vi "JL_Get_Latest_Build_From_Artifactory.vi"(0 "Repository":string="CIBuild", 11 "Error In":errorcluster) -> (4 "Output Path":path, 6 "Build":string, 15 "Error Out":errorcluster)   [LabVIEW 2019]
uses:
  <vilib>/regexp/Match Regular Expression.xnode
  <vilib>/httpClient/LabVIEWHTTPClient.lvlib
  <vilib>/zip/NI_Unzip.lvlib
panel:
  out "Numeric":i32
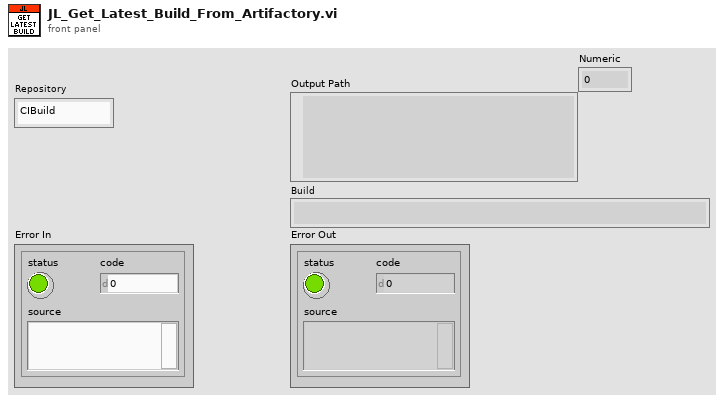
[diagram p1: front panel]
types:
  T1 = typedef "LabVIEWHTTPClient.lvlib/ClientHandle.ctl" = refnum<k1>
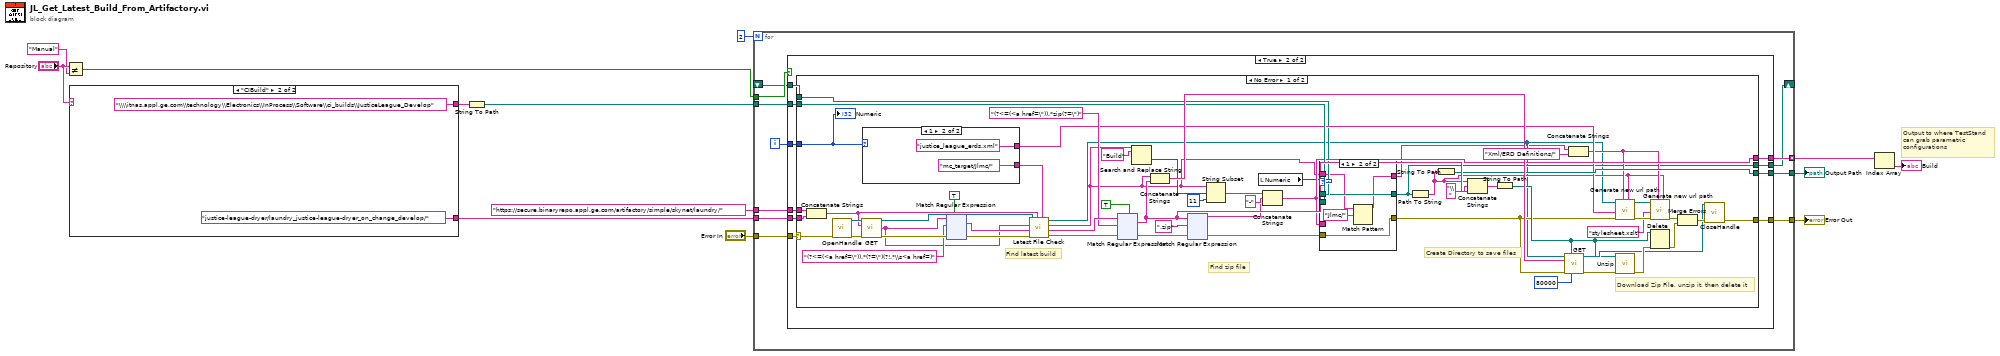
[diagram p0: block diagram]
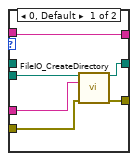
[diagram p3: hidden frame]
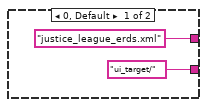
[diagram p4: hidden frame]
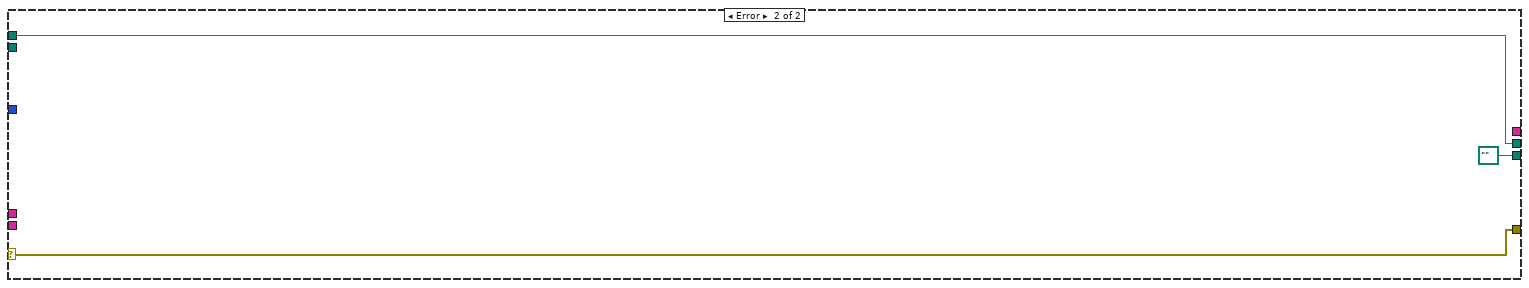
[diagram p5: hidden frame]
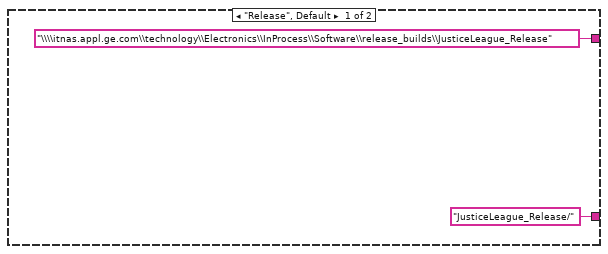
[diagram p6: hidden frame]
diagram:
  # "Output to where TestStand\ncan grab parametric\nconfigurations"
  n1 = Not Equal?(x="Repository", y="Manual") -> (x != y?=w12:bool)
  n2 = case shown="\"CIBuild\"" "Repository" {
    tunnel: ["\\\\itnas.appl.ge.com\\technology\\Electronics\\InProcess\\Software\\release_builds\\JusticeLeague_Release" "\\\\itnas.appl.ge.com\\technology\\Electronics\\InProcess\\Software\\ci_builds\\JusticeLeague_Develop"] -> w13
    tunnel: ["JusticeLeague_Release/" "justice-league-dryer/laundry_justice-league-dryer_on_change_develop/"] -> w9
    frame "Release", Default {
    }
    frame "CIBuild" {
    }
  }
  n3 = String To Path(string=w13) -> (path=w8:path)
  n4 = for {
    N: 2 -> [_]
    tunnel: w12 -> [w28]
    tunnel: w9 -> [w27]
    tunnel: w8 -> [w26]
    tunnel: [w25] -> w7
    tunnel: "https://secure.binaryrepo.appl.ge.com/artifactory/simple/skynet/laundry/" ("regular expression") -> [w24]
    tunnel: [w23] -> w2 mode=indexing
    tunnel: [w22] -> w5
    tunnel: "Error In" -> [w21]
    shift-right: [w19] -> _
    shift-left: _ -> [w18]
    i -> [w20]
    n5 = case shown="True" w28 {
      tunnel: w24 -> [_ w40]
      tunnel: [_ w39] -> w25
      tunnel: [w30 w38] -> w22
      tunnel: w26 -> [_ w37]
      tunnel: w27 -> [_ w36]
      tunnel: [_ w35] -> w23
      tunnel: w21 -> [w30 w34]
      tunnel: w20 -> [_ w33]
      tunnel: [w29 w32] -> w19
      tunnel: w18 -> [w29 w31]
      frame False {
      }
      frame True {
        n6 = case shown="No Error" w34 {
          selector: w34 -> [w61 w458]
          tunnel: [w65 w458] -> w38
          tunnel: [w76 path ""] -> w39
          tunnel: w36 -> [w93 _]
          tunnel: w40 -> [w94 _]
          tunnel: w37 -> [w77 _]
          tunnel: [w62 _] -> w35
          tunnel: w33 -> [w53 _]
          tunnel: [w49 w456] -> w32
          tunnel: w31 -> [w48 w456]
          frame No Error {
            # "Find latest build"
            # "Create Directory to save files"
            # "Find zip file"
            # "Download Zip File, unzip it, then delete it"
            n7 = Concatenate Strings(w94, w93) -> (w95:string)
            n8 = call <vilib>:"OpenHandle.vi"("error in (no error)"=w61) -> ("client handle out"=w97:T1, "error out"=w98:errorcluster)  [unwired: 13 in]
            n9 = call <vilib>:"GET.vi"("client handle"=w97, "url"=w95, "error in (no error)"=w98) -> ("client handle out"=w46:T1, "body"=w43:string, "error out"=w96:errorcluster)  [unwired: 9 in, 1 out]
            n10 = case shown="1" w53 {
              tunnel: ["ui_target/" ("string") "mc_target/Jlmc/" ("string")] -> w74
              tunnel: ["justice_league_erds.xml" ("regular expression") "justice_league_erds.xml" ("regular expression")] -> w60
              frame 0, Default {
              }
              frame 1 {
              }
            }
            n11 = xnode "Match Regular Expression"("input string"=w43, "regular expression"="(?<=(<a href=\")).*(?=\")(?!.*\\s<a href=)", "error in"=w96, "multiline? (F)"=TRUE) -> ("whole match"=w44:string, "error out"=w90:errorcluster)  [unwired: 2 in, 3 out]
            n12 = call "Latest File Check.vi"("Target File Path"=w74, "Initial File Path"=w95, "error in (no error)"=w90, "Matched Folder"=w44, "Initial body in"=w43, "Refnum in"=w46) -> ("error out"=w88:errorcluster, "body out"=w87:string, "File Path Out"=w42:string, "Refnum out"=w45:T1)  [unwired: 2 in]
            n13 = xnode "Match Regular Expression"("input string"=w87, "regular expression"="(?<=(<a href=\")).*zip(?=\")", "error in"=w88, "multiline? (F)"=TRUE) -> ("whole match"=w81:string, "error out"=w83:errorcluster)  [unwired: 2 in, 3 out]
            n14 = Search and Replace String(input string=w42, search string="Build") -> (offset past replacement=w71:i32)  [unwired: 6 in, 3 out]
            n15 = Concatenate Strings(w42, w81) -> (w85:string)
            n16 = xnode "Match Regular Expression"("input string"=w81, "regular expression"=".zip", "error in"=w83) -> ("before match"=w68:string, "error out"=w82:errorcluster)  [unwired: 3 in, 3 out]
            n17 = String Subset(string=w42, offset (0)=w71, length (rest)=11 ("length (rest)")) -> (substring=w70:string)
            n18 = local read "Numeric"() -> (w50:i32)
            n19 = Concatenate Strings(w70, "-" ("string"), w68) -> (w62:string)
            n20 = case shown="1" w50 {
              tunnel: [w104 w108] -> w47
              tunnel: w82 -> [w103 w108]
              tunnel: w77 -> [w102 _]
              tunnel: [w101 w109] -> w49
              tunnel: w62 -> [w100 _]
              tunnel: w48 -> [_ w109]
              tunnel: w42 -> [w99 w106]
              tunnel: [w99 w107] -> w41
              frame 0, Default {
                n21 = call "FileIO_CreateDirectory.vi"("Base Path"=w102, "Directory Name"=w100, "Error In"=w103) -> ("File Path Control"=w101:path, "Error Out"=w104:errorcluster)  [unwired: 11 in]
              }
              frame 1 {
                n22 = Match Pattern(string=w106, regular expression="Jlmc/") -> (before substring=w107:string)  [unwired: 1 in, 3 out]
              }
            }
            n23 = Path To String(path=w49) -> (string=w54:string)
            n24 = String To Path(string=w54) -> (path=w76:path)
            n25 = Concatenate Strings(w54, "\\" ("string"), w81) -> (w79:string)
            n26 = String To Path(string=w79) -> (path=w51:path)
            n27 = call <vilib>:"GET.vi"("client handle"=w45, "output file"=w51, "url"=w85, "error in (no error)"=w47, "timeout (10000)"=80000) -> ("client handle out"=w63:T1, "error out"=w64:errorcluster)  [unwired: 7 in, 2 out]
            n28 = Concatenate Strings(w41, "Xml/ERD Definitions/" ("string")) -> (w57:string)
            n29 = call "Generate new url path.vi"("Input Path string"=w54, "Appending File Path"=w57, "error in (no error)"=w47, "Style/ERD"=w60, "Refnum"=w45) -> ("error out"=w59:errorcluster, "Ref out"=w56:T1)  [unwired: 5 in]
            n30 = call <vilib>:"Unzip.vi"("error in (no error)"=w64, "Zip file"=w51) -> ("error out"=w78:errorcluster)  [unwired: 7 in, 2 out]
            n31 = call "Generate new url path.vi"("Input Path string"=w54, "Appending File Path"=w57, "error in (no error)"=w59, "Style/ERD"="stylesheet.xslt" ("regular expression"), "Refnum"=w56) -> ("error out"=w58:errorcluster)  [unwired: 5 in, 1 out]
            n32 = Delete(path (use dialog)=w51, error in=w78) -> (error out=w67:errorcluster)  [unwired: 3 in, 2 out]
            n33 = Merge Errors(w58, w67) -> (w66:errorcluster)
            n34 = call <vilib>:"CloseHandle.vi"("client handle"=w63, "error in (no error)"=w66) -> ("error out"=w65:errorcluster)  [unwired: 13 in]
            "Numeric" <- w53
          }
          frame Error {
          }
        }
      }
    }
  }
  "Output Path" <- w7
  "Error Out" <- w5
  n35 = Index Array(array=w2) -> (element=→"Build":string)  [unwired: 1 in]
